vi "Drive_Hardware_Swerve_Module.vi"(5 "Drive Invert Type":T2, 6 "Module Name":string, 7 "error in":errorcluster, 8 "Encoder CAN ID":u8, 9 "Azimuth CAN ID":u8, 10 "Drive CAN ID":u8) -> (0 "error out":errorcluster)   [LabVIEW 2020]
uses:
  <vilib>/Rock Robotics/WPI/ThirdParty/Phoenix-LabVIEW/Motor Controller/Controls/CTRE_Phoenix_MotorControl_TalonFXInvertType.ctl
  <vilib>/Rock Robotics/WPI/ThirdParty/Phoenix-LabVIEW/Motor Controller/Controls/CTRE_Phoenix_MotorControl_SupplyCurrentLimitConfiguration.ctl
  <vilib>/Rock Robotics/WPI/ThirdParty/Phoenix-LabVIEW/Motor Controller/Controls/CTRE_Phoenix_MotorControl_NeutralMode.ctl
  <vilib>/Rock Robotics/WPI/ThirdParty/Phoenix-LabVIEW/CANCoder/Controls/CTRE_Phoenix_CANcoder_StatusFrame.ctl
  <vilib>/Rock Robotics/WPI/ThirdParty/Phoenix-LabVIEW/CANCoder/Controls/CTRE_Phoenix_CANcoder_SensorInitializationStrategy.ctl
panel:
  in  "Azimuth Current Limits":T1={"Enable?"=TRUE, "Current Limit"=30.0, "Threshold Current"=0.0, "Threshold Time"=0.0}
  in  "Drive Current Limits":T1={"Enable?"=TRUE, "Current Limit"=40.0, "Threshold Current"=0.0, "Threshold Time"=0.0}
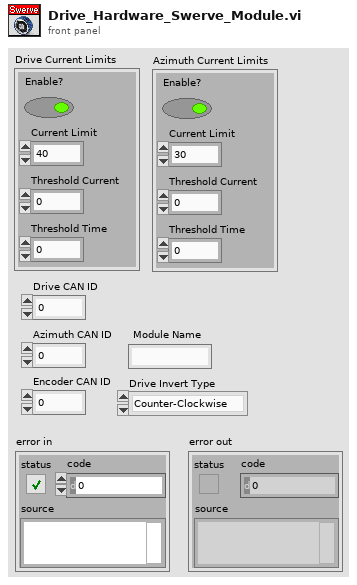
[diagram p1: front panel]
types:
  T1 = typedef "CTRE_Phoenix_MotorControl_SupplyCurrentLimitConfiguration.ctl" = cluster{"Enable?":bool, "Current Limit":dbl, "Threshold Current":dbl, "Threshold Time":dbl}
  T2 = typedef "CTRE_Phoenix_MotorControl_TalonFXInvertType.ctl" = enum16{"Counter-Clockwise", "Clockwise"}
  T3 = typedef "WPI_MotorControlDeviceRef.ctl" = cluster{"DeviceStatus":errorcluster, "Type":T4, "PWM":cluster{"PWM Channel":T5, "DeadBand":T6}, "CAN":cluster{"Device Number":u8, "SetOutput VI Ref":variant, "GetOutput VI Ref":variant, "Enable VI Ref":variant, "Disable VI Ref":variant, "Data":variant}, "Invert":bool, "DIO PWM":cluster{"PWM \"Enable\" Channel":T5, "DIOChannel":T7, "PWM Rate":dbl}}
  T4 = typedef "WPI_MotorControlType.ctl" = enum16{"PWM", "CAN", "DIO PWM"}
  T5 = typedef "FPGA_DIOPWMChannel.ctl" = enum8{"PWM 0", "PWM 1", "PWM 2", "PWM 3", "PWM 4", "PWM 5", "PWM 6", "PWM 7", "PWM 8", "PWM 9", "PWM MXP 0", "PWM MXP 1", "PWM MXP 2", "PWM MXP 3", "PWM MXP 4", "PWM MXP 5", "PWM MXP 6", "PWM MXP 7", "PWM MXP 8", "PWM MXP 9", "Invalid"}
  T6 = typedef "WPI_PWMDeadband.ctl" = cluster{"Name":string, "maxPositivePwm":i32, "minPositivePwm":i32, "centerPwm":i32, "maxNegativePwm":i32, "minNegativePwm":i32, "angularRange":u16}
  T7 = typedef "FPGA_DIOChannel.ctl" = enum8{"DIO 0", "DIO 1", "DIO 2", "DIO 3", "DIO 4", "DIO 5", "DIO 6", "DIO 7", "DIO 8", "DIO 9", "DIO MXP 0", "DIO MXP 1", "DIO MXP 2", "DIO MXP 3", "DIO MXP 4", "DIO MXP 5", "DIO MXP 6", "DIO MXP 7", "DIO MXP 8", "DIO MXP 9", "DIO MXP 10", "DIO MXP 11", "DIO MXP 12", "DIO MXP 13", "DIO MXP 14", "DIO MXP 15", "SPI Port CS1", "SPI Port CS2", "SPI Port CS3", "SPI Port MISO", "SPI Port MOSI", "Invalid"}
  T8 = typedef "CTRE_Phoenix_MotorControl_NeutralMode.ctl" = enum8{"EEPROMSetting", "Override to Coast", "Override to Brake"}
  T9 = typedef "CTRE_Phoenix_CANcoder_DeviceRef.ctl" = cluster{"DeviceStatus":errorcluster, "Device Number":u8, "Handle":u64, "UsageFrame":u32, "Library Path":path}
  T10 = typedef "CTRE_Phoenix_CANcoder_StatusFrame.ctl" = u32
  T11 = typedef "CTRE_Phoenix_CANcoder_SensorInitializationStrategy.ctl" = enum16{"Boot To Zero", "Boot To Absolute Position"}
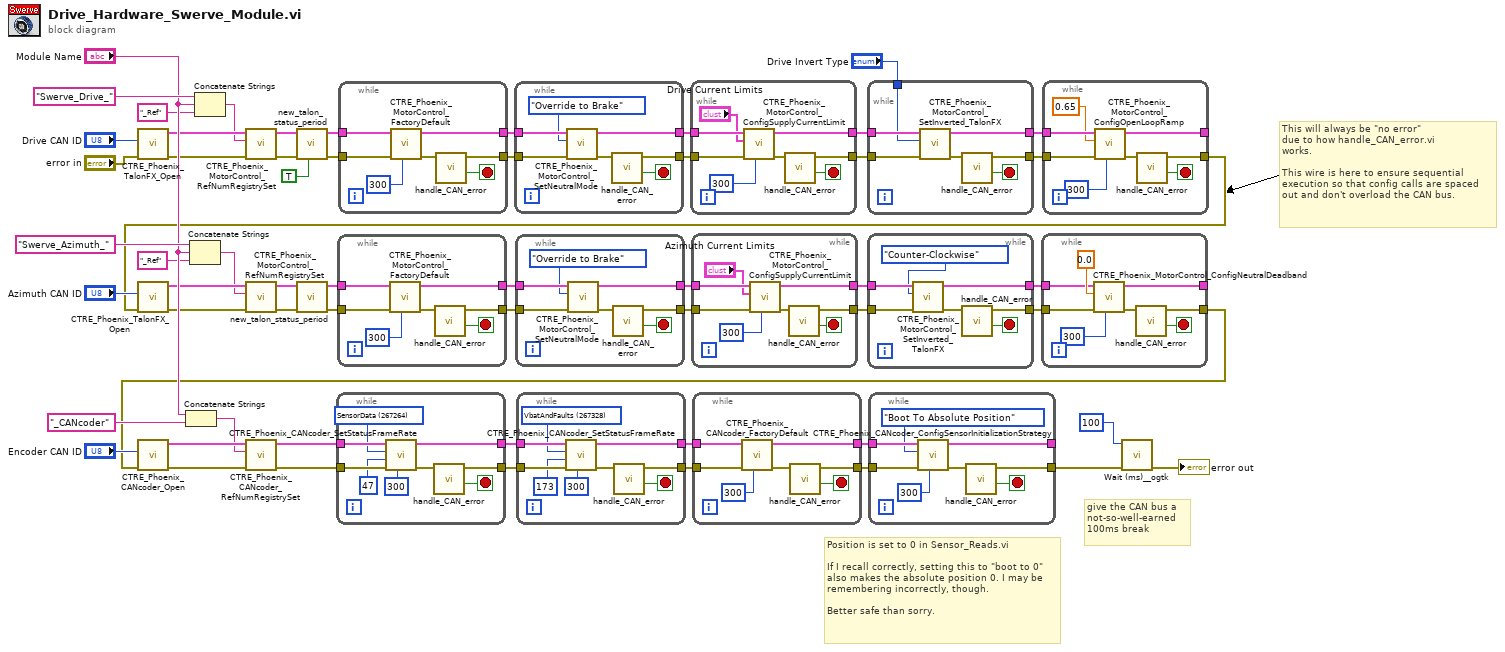
[diagram p0: block diagram]
diagram:
  # "Position is set to 0 in Sensor_Reads.vi\n\nIf I recall correctly, setting this to \"boot to 0\"\nalso makes the absolute position 0. I may be\nremembering incorrectly, though.\n\nBetter safe than sorry."
  # "This will always be \"no error\"\ndue to how handle_CAN_error.vi\nworks.\n\nThis wire is here to ensure sequential\nexecution so that config calls are spaced\nout and don't overload the CAN bus."
  # "give the CAN bus a\nnot-so-well-earned\n100ms break"
  n1 = call <vilib>:"CTRE_Phoenix_TalonFX_Open.vi"("error in"="error in", "Device Number"="Drive CAN ID") -> ("error out"=w27:errorcluster, "PhoenixMotorControlDevRef"=w26:T3)  [unwired: 8 in]
  n2 = Concatenate Strings("Module Name", "_CANcoder" ("string")) -> (w22:string)
  n3 = Concatenate Strings("Swerve_Azimuth_" ("string"), "Module Name", "_Ref" ("string")) -> (w23:string)
  n4 = Concatenate Strings("Swerve_Drive_" ("string"), "Module Name", "_Ref" ("string")) -> (w24:string)
  n5 = call <vilib>:"CTRE_Phoenix_MotorControl_RefNumRegistrySet.vi"("error in (no error)"=w27, "refnum name"=w24, "PhoenixMotorControlDevRef"=w26) -> ("error out"=w16:errorcluster, "PhoenixMotorControlDevRef"=w15:T3)  [unwired: 7 in]
  n6 = call "new_talon_status_period.vi"("Feedback Data?"=TRUE, "error in (no error)"=w16, "PhoenixMotorControlDevRef"=w15) -> ("error out"=w52:errorcluster, "PhoenixMotorControlDevRef"=w53:T3)  [unwired: 7 in]
  n7 = while {
    tunnel: w53 -> [w64]
    tunnel: w52 -> [w61]
    tunnel: [w60] -> w51
    tunnel: [w59] -> w48
    stop <- w62 stop-if-true
    n8 = call <vilib>:"CTRE_Phoenix_MotorControl_FactoryDefault.vi"("timeoutMs"=300, "error in"=w61, "PhoenixMotorControlDevRef"=w64) -> ("error out"=w63:errorcluster, "PhoenixMotorControlDevRef"=w60:T3)  [unwired: 7 in]
    n9 = call "handle_CAN_error.vi"("error in (no error)"=w63) -> ("stop"=w62:bool, "error out"=w59:errorcluster)  [unwired: 9 in]
  }
  n10 = while {
    tunnel: w51 -> [w72]
    tunnel: w48 -> [w69]
    tunnel: [w68] -> w50
    tunnel: [w67] -> w49
    stop <- w70 stop-if-true
    n11 = call <vilib>:"CTRE_Phoenix_MotorControl_SetNeutralMode.vi"("error in (no error)"=w69, "Motor Control Neutral Mode"=CTRE_Phoenix_MotorControl_NeutralMode."Override to Brake", "PhoenixMotorControlDevRef"=w72) -> ("error out"=w71:errorcluster, "PhoenixMotorControlDevRef"=w68:T3)  [unwired: 7 in]
    n12 = call "handle_CAN_error.vi"("error in (no error)"=w71) -> ("stop"=w70:bool, "error out"=w67:errorcluster)  [unwired: 9 in]
  }
  n13 = while {
    tunnel: [w80] -> w12
    tunnel: [w78] -> w11
    tunnel: w50 -> [w77]
    tunnel: w49 -> [w76]
    stop <- w79 stop-if-true
    n14 = call <vilib>:"CTRE_Phoenix_MotorControl_ConfigSupplyCurrentLimit.vi"("timeoutMs"=u32 300, "error in (no error)"=w76, "Supply Current Limit Configuration"="Drive Current Limits", "PhoenixMotorControlDevRef"=w77) -> ("error out"=w73:errorcluster, "PhoenixMotorControlDevRef"=w78:T3)  [unwired: 6 in]
    n15 = call "handle_CAN_error.vi"("error in (no error)"=w73) -> ("stop"=w79:bool, "error out"=w80:errorcluster)  [unwired: 9 in]
  }
  n16 = while {
    tunnel: [w85] -> w13
    tunnel: [w87] -> w14
    tunnel: w11 -> [w83]
    tunnel: w12 -> [w82]
    tunnel: "Drive Invert Type" -> [w81]
    stop <- w84 stop-if-true
    n17 = call <vilib>:"CTRE_Phoenix_MotorControl_SetInverted_TalonFX.vi"("error in (no error)"=w82, "Invert Type"=w81, "PhoenixMotorControlDevRef"=w83) -> ("error out"=w86:errorcluster, "PhoenixMotorControlDevRef"=w87:T3)  [unwired: 7 in]
    n18 = call "handle_CAN_error.vi"("error in (no error)"=w86) -> ("stop"=w84:bool, "error out"=w85:errorcluster)  [unwired: 9 in]
  }
  n19 = while {
    tunnel: [w93] -> w4
    tunnel: [w95] -> _
    tunnel: w14 -> [w91]
    tunnel: w13 -> [w90]
    stop <- w92 stop-if-true
    n20 = call <vilib>:"CTRE_Phoenix_MotorControl_ConfigOpenLoopRamp.vi"("timeoutMs"=u32 300, "error in (no error)"=w90, "secondsFromNeutralToFull"=0.65, "PhoenixMotorControlDevRef"=w91) -> ("error out"=w94:errorcluster, "PhoenixMotorControlDevRef"=w95:T3)  [unwired: 6 in]
    n21 = call "handle_CAN_error.vi"("error in (no error)"=w94) -> ("stop"=w92:bool, "error out"=w93:errorcluster)  [unwired: 9 in]
  }
  n22 = call <vilib>:"CTRE_Phoenix_TalonFX_Open.vi"("error in"=w4, "Device Number"="Azimuth CAN ID") -> ("error out"=w29:errorcluster, "PhoenixMotorControlDevRef"=w28:T3)  [unwired: 8 in]
  n23 = call <vilib>:"CTRE_Phoenix_MotorControl_RefNumRegistrySet.vi"("error in (no error)"=w29, "refnum name"=w23, "PhoenixMotorControlDevRef"=w28) -> ("error out"=w17:errorcluster, "PhoenixMotorControlDevRef"=w18:T3)  [unwired: 7 in]
  n24 = call "new_talon_status_period.vi"("error in (no error)"=w17, "PhoenixMotorControlDevRef"=w18) -> ("error out"=w46:errorcluster, "PhoenixMotorControlDevRef"=w47:T3)  [unwired: 8 in]
  n25 = while {
    tunnel: w47 -> [w101]
    tunnel: w46 -> [w98]
    tunnel: [w97] -> w45
    tunnel: [w96] -> w44
    stop <- w99 stop-if-true
    n26 = call <vilib>:"CTRE_Phoenix_MotorControl_FactoryDefault.vi"("timeoutMs"=300, "error in"=w98, "PhoenixMotorControlDevRef"=w101) -> ("error out"=w100:errorcluster, "PhoenixMotorControlDevRef"=w97:T3)  [unwired: 7 in]
    n27 = call "handle_CAN_error.vi"("error in (no error)"=w100) -> ("stop"=w99:bool, "error out"=w96:errorcluster)  [unwired: 9 in]
  }
  n28 = while {
    tunnel: w45 -> [w109]
    tunnel: w44 -> [w106]
    tunnel: [w105] -> w10
    tunnel: [w104] -> w9
    stop <- w107 stop-if-true
    n29 = call <vilib>:"CTRE_Phoenix_MotorControl_SetNeutralMode.vi"("error in (no error)"=w106, "Motor Control Neutral Mode"=CTRE_Phoenix_MotorControl_NeutralMode."Override to Brake", "PhoenixMotorControlDevRef"=w109) -> ("error out"=w108:errorcluster, "PhoenixMotorControlDevRef"=w105:T3)  [unwired: 7 in]
    n30 = call "handle_CAN_error.vi"("error in (no error)"=w108) -> ("stop"=w107:bool, "error out"=w104:errorcluster)  [unwired: 9 in]
  }
  n31 = while {
    tunnel: [w115] -> w7
    tunnel: [w117] -> w8
    tunnel: w10 -> [w113]
    tunnel: w9 -> [w112]
    stop <- w114 stop-if-true
    n32 = call <vilib>:"CTRE_Phoenix_MotorControl_ConfigSupplyCurrentLimit.vi"("timeoutMs"=u32 300, "error in (no error)"=w112, "Supply Current Limit Configuration"="Azimuth Current Limits", "PhoenixMotorControlDevRef"=w113) -> ("error out"=w116:errorcluster, "PhoenixMotorControlDevRef"=w117:T3)  [unwired: 6 in]
    n33 = call "handle_CAN_error.vi"("error in (no error)"=w116) -> ("stop"=w114:bool, "error out"=w115:errorcluster)  [unwired: 9 in]
  }
  n34 = while {
    tunnel: [w124] -> w5
    tunnel: [w120] -> w6
    tunnel: w8 -> [w122]
    tunnel: w7 -> [w121]
    stop <- w123 stop-if-true
    n35 = call <vilib>:"CTRE_Phoenix_MotorControl_SetInverted_TalonFX.vi"("error in (no error)"=w121, "Invert Type"=CTRE_Phoenix_MotorControl_TalonFXInvertType."Counter-Clockwise" ("Drive Invert Type"), "PhoenixMotorControlDevRef"=w122) -> ("error out"=w119:errorcluster, "PhoenixMotorControlDevRef"=w120:T3)  [unwired: 7 in]
    n36 = call "handle_CAN_error.vi"("error in (no error)"=w119) -> ("stop"=w123:bool, "error out"=w124:errorcluster)  [unwired: 9 in]
  }
  n37 = while {
    tunnel: [w129] -> w3
    tunnel: [w131] -> _
    tunnel: w6 -> [w127]
    tunnel: w5 -> [w126]
    stop <- w128 stop-if-true
    n38 = call <vilib>:"CTRE_Phoenix_MotorControl_ConfigNeutralDeadband.vi"("timeoutMs"=u32 300, "error in (no error)"=w126, "Percent Deadband"=0.0 ("Saturation Voltage"), "PhoenixMotorControlDevRef"=w127) -> ("error out"=w130:errorcluster, "PhoenixMotorControlDevRef"=w131:T3)  [unwired: 6 in]
    n39 = call "handle_CAN_error.vi"("error in (no error)"=w130) -> ("stop"=w128:bool, "error out"=w129:errorcluster)  [unwired: 9 in]
  }
  n40 = call <vilib>:"CTRE_Phoenix_CANcoder_Open.vi"("error in"=w3, "Device Number"="Encoder CAN ID") -> ("error out"=w30:errorcluster, "CTRE_CANcoder_DeviceRef"=w31:T9)  [unwired: 8 in]
  n41 = call <vilib>:"CTRE_Phoenix_CANcoder_RefNumRegistrySet.vi"("error in (no error)"=w30, "refnum name"=w22, "CTRE_CANcoder_DeviceRef"=w31) -> ("error out"=w19:errorcluster, "CTRE_CANcoder_DeviceRef"=w20:T9)  [unwired: 7 in]
  n42 = while {
    tunnel: w20 -> [w139]
    tunnel: w19 -> [w138]
    tunnel: [w133] -> w42
    tunnel: [w140] -> w41
    stop <- w141 stop-if-true
    w136 = T10 267264 items=["SensorData"=267264, "VbatAndFaults"=267328] ("CANcoder Status Frame")
    n43 = call <vilib>:"CTRE_Phoenix_CANcoder_SetStatusFrameRate.vi"("timeoutMs"=u32 300, "error in (no error)"=w138, "Period (ms)"=u8 47, "CANcoder Status Frame"=w136, "CTRE_CANcoder_DeviceRef"=w139) -> ("error out"=w134:errorcluster, "CTRE_CANcoder_DeviceRef"=w133:T9)  [unwired: 5 in]
    n44 = call "handle_CAN_error.vi"("error in (no error)"=w134) -> ("stop"=w141:bool, "error out"=w140:errorcluster)  [unwired: 9 in]
  }
  n45 = while {
    tunnel: w42 -> [w148]
    tunnel: w41 -> [w147]
    tunnel: [w142] -> w40
    tunnel: [w149] -> w39
    stop <- w150 stop-if-true
    w145 = T10 267328 items=["SensorData"=267264, "VbatAndFaults"=267328] ("CANcoder Status Frame")
    n46 = call <vilib>:"CTRE_Phoenix_CANcoder_SetStatusFrameRate.vi"("timeoutMs"=u32 300, "error in (no error)"=w147, "Period (ms)"=u8 173, "CANcoder Status Frame"=w145, "CTRE_CANcoder_DeviceRef"=w148) -> ("error out"=w143:errorcluster, "CTRE_CANcoder_DeviceRef"=w142:T9)  [unwired: 5 in]
    n47 = call "handle_CAN_error.vi"("error in (no error)"=w143) -> ("stop"=w150:bool, "error out"=w149:errorcluster)  [unwired: 9 in]
  }
  n48 = while {
    tunnel: w40 -> [w155]
    tunnel: w39 -> [w154]
    tunnel: [w152] -> w37
    tunnel: [w156] -> w36
    stop <- w157 stop-if-true
    n49 = call <vilib>:"CTRE_Phoenix_CANcoder_FactoryDefault.vi"("timeoutMs"=300, "error in"=w154, "CTRE_CANcoder_DeviceRef"=w155) -> ("error out"=w153:errorcluster, "CTRE_CANcoder_DeviceRef"=w152:T9)  [unwired: 7 in]
    n50 = call "handle_CAN_error.vi"("error in (no error)"=w153) -> ("stop"=w157:bool, "error out"=w156:errorcluster)  [unwired: 9 in]
  }
  n51 = while {
    tunnel: w37 -> [w163]
    tunnel: w36 -> [w162]
    tunnel: [w160] -> _
    tunnel: [w164] -> w2
    stop <- w165 stop-if-true
    n52 = call <vilib>:"CTRE_Phoenix_CANcoder_ConfigSensorInitializationStrategy.vi"("timeoutMs"=300, "error in"=w162, "Sensor Initialization Strategy"=CTRE_Phoenix_CANcoder_SensorInitializationStrategy."Boot To Absolute Position", "CTRE_CANcoder_DeviceRef"=w163) -> ("error out"=w161:errorcluster, "CTRE_CANcoder_DeviceRef"=w160:T9)  [unwired: 6 in]
    n53 = call "handle_CAN_error.vi"("error in (no error)"=w161) -> ("stop"=w165:bool, "error out"=w164:errorcluster)  [unwired: 9 in]
  }
  n54 = call "Wait (ms)__ogtk.vi"("error in (no error)"=w2, "milliseconds to wait"=u32 100) -> ("error out"=→"error out":errorcluster)  [unwired: 8 in, 1 out]
